vi "Get bronkhorst param from PGserver.vi"(6 "conninfo":T2={"host"="localhost", "port"="5432", "client_encoding"="WIN1251", "dbname"="data", "user"="postgres", "password"=""}, 8 "error in (no error)":errorcluster, 9 "RegParamColumns":string[](array[string])=["instrument_range_max", "auto_value", "alr_value", "output_k", "output_set_time", "group", "process_units", "process_gas", "fcode", "fcode_full", "shortname"], 10 "AIParamTable":string="bronkhorst", 11 "AIParameters":string[](array[string])) -> (0 "error out":errorcluster, 2 "Names table":string[][](array[string]), 3 "Parameters table":dbl[][](array[numeric]))   [LabVIEW 2019, in "control.lvlib"]
uses:
  control.lvlib
  Database/ctl/Coninfo.ctl
  Database/PostgreSQL2LabVIEW/libpqlv/src/PQfinish.vi
  Database/PostgreSQL2LabVIEW/libpqlv/src/PQconnectdb.vi
  Database/PostgreSQL2LabVIEW/libpqlv/src/PQerrorMessage.vi
  Database/PostgreSQL2LabVIEW/libpqlv/src/PQstatus.vi
  <vilib>/dlg_ctls.llb/Space Constant.vi
  Database/Progress.vi
  Database/PostgreSQL.lvlib
  Database/PostgreSQL2LabVIEW/libpqUtility64/libpqutility64.lvlib
  Database/PostgreSQL2LabVIEW/libpqUtility/libpqutility.lvlib
panel:
  out "PQStatus":T1(ring)
  # "group"
  # "process_gas"
  # "fcode"
  # "fcode_full"
  # "shortname"
  # "instrument_range_max"
  # "auto_value"
  # "alr_value"
  # "output_k"
  # "output_set_time"
  # "process_units"
  # "Names"
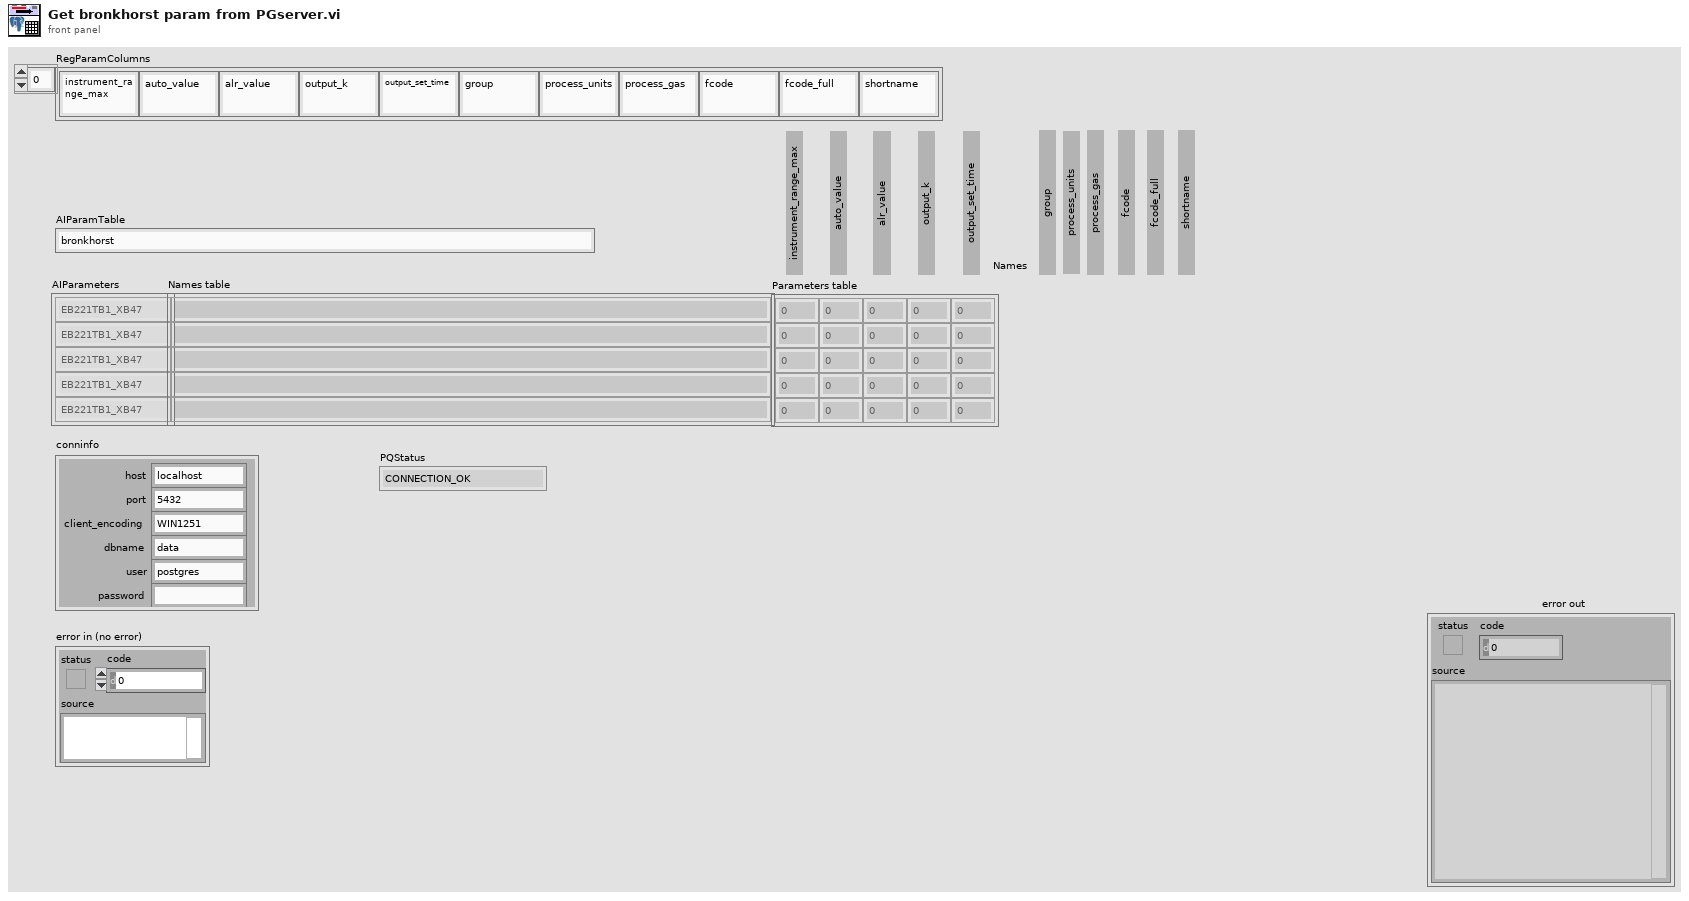
[diagram p1: front panel]
types:
  T1 = enum32{"CONNECTION_OK", "CONNECTION_BAD", "CONNECTION_STARTED", "CONNECTION_MADE", "CONNECTION_AWAITING_RESPONSE", "CONNECTION_AUTH_OK", "CONNECTION_SETENV", "CONNECTION_SSL_STARTUP", "CONNECTION_NEEDED"}
  T2 = typedef "PostgreSQL.lvlib/Coninfo.ctl" = cluster{"host":string, "port":string, "client_encoding":string, "dbname":string, "user":string, "password":string}
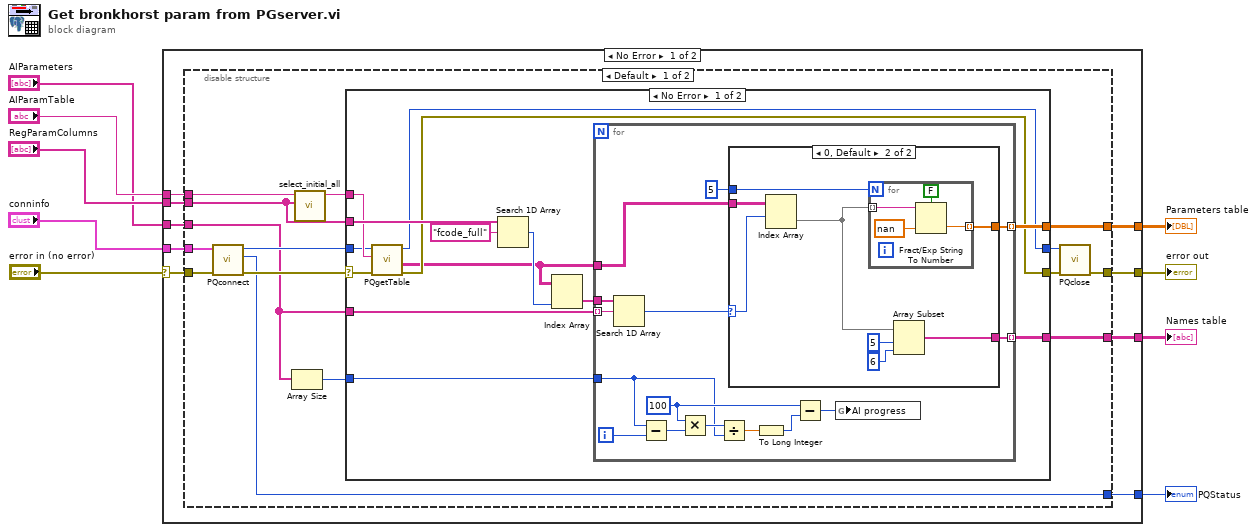
[diagram p0: block diagram]
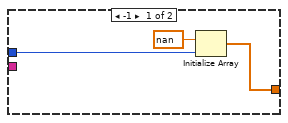
[diagram p2: hidden frame]
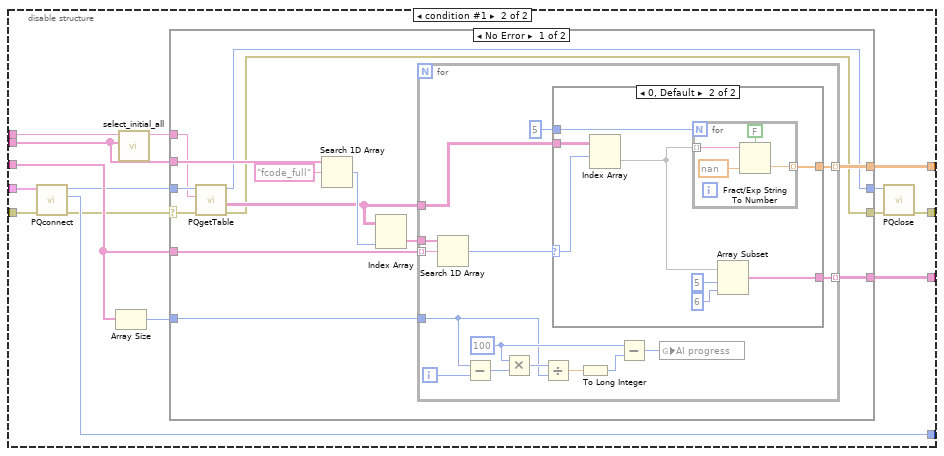
[diagram p4: hidden frame]
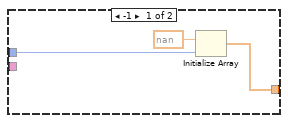
[diagram p5: hidden frame]
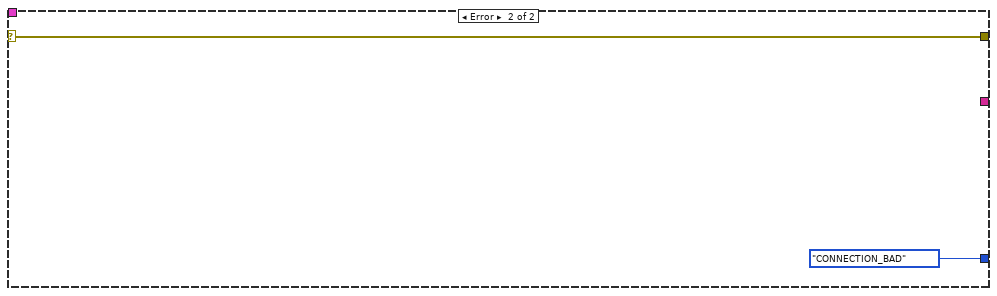
[diagram p7: hidden frame]
diagram:
  n1 = case shown="No Error" "error in (no error)" {
    selector: "error in (no error)" -> [w17 w142]
    tunnel: [w12 w142] -> w9
    tunnel: [w13 _] -> w8
    tunnel: [w11 _] -> w7
    tunnel: "RegParamColumns" -> [w15 _]
    tunnel: "conninfo" -> [w18 _]
    tunnel: "AIParamTable" -> [w16 _]
    tunnel: "AIParameters" -> [w14 _]
    tunnel: [w10 T1."CONNECTION_BAD" ("PQStatus")] -> w1
    frame No Error {
      n2 = disable-structure shown="Default" {
        disable-tunnel: [w22 w80] -> w12
        disable-tunnel: [w27 w88] -> w13
        disable-tunnel: [w26 w89] -> w11
        disable-tunnel: w15 -> [w19 w91]
        disable-tunnel: w18 -> [w30 w87]
        disable-tunnel: w16 -> [w21 w92]
        disable-tunnel: w14 -> [w28 w90]
        disable-tunnel: w17 -> [w29 w86]
        disable-tunnel: [w25 w84] -> w10
        frame condition #0 (active) {
          n3 = call "PQconnect.vi"("error in (no error)"=w29, "conninfo"=w30) -> ("error out"=w33:errorcluster, "PQStatus"=w25:T1, "conn"=w32:u32)  [unwired: 7 in]
          n4 = Array Size(array=w28) -> (size(s)=w31:i32)
          n5 = call "select_initial_all.vi"("Column table"=w19, "table"=w21) -> ("parameters"=w20:string)  [unwired: 8 in, 1 out]
          n6 = case shown="No Error" w33 {
            selector: w33 -> [w40 w79]
            tunnel: w28 -> [w34 _]
            tunnel: [w47 _] -> w27
            tunnel: [w46 _] -> w26
            tunnel: w31 -> [w45 _]
            tunnel: w32 -> [w38 w78]
            tunnel: w20 -> [w39 _]
            tunnel: [w37 w79] -> w23
            tunnel: [w36 w78] -> w24
            tunnel: w19 -> [w41 _]
            frame No Error {
              n7 = call "PQgetTable.vi"("error in"=w40, "query"=w39, "conn"=w38) -> ("error out"=w37:errorcluster, "Data"=w35:string[][], "conn_out"=w36:u32)  [unwired: 4 in, 2 out]
              n8 = Search 1D Array(1D array=w41, element="fcode_full" ("table")) -> (index of element=w43:i32)  [unwired: 1 in]
              n9 = Index Array(array=w35, index (col)=w43) -> (element=w42:string[])  [unwired: 1 in]
              n10 = for {
                tunnel: [w62] -> w46 mode=indexing
                tunnel: [w61] -> w47 mode=indexing
                tunnel: w45 -> [w53]
                tunnel: w42 -> [w51]
                tunnel: w35 -> [w50]
                tunnel: w34 -> [w49] mode=indexing
                i -> [w54]
                w58 = 100 ("y")
                n11 = Search 1D Array(1D array=w51, element=w49) -> (index of element=w48:i32)  [unwired: 1 in]
                n12 = Subtract(x=w53, y=w54) -> (x-y=w57:i32)
                n13 = Multiply(x=w58, y=w57) -> (x*y=w60:i32)
                n14 = Divide(x=w60, y=w53) -> (x/y=w56:dbl)
                n15 = case shown="0, Default" w48 {
                  selector: w48 -> [_ w68]
                  tunnel: [w64 w67] -> w61
                  tunnel: 5 ("y") -> [w63 w71]
                  tunnel: w50 -> [_ w70]
                  tunnel: [_ w72] -> w62
                  frame -1 {
                    n16 = Initialize Array(nan, w63) -> (w64:dbl[])
                  }
                  frame 0, Default {
                    n17 = Index Array(array=w70, index (row)=w68) -> (element=w69:string[])  [unwired: 1 in]
                    n18 = for {
                      N: w71 -> [_]
                      tunnel: w69 -> [w76] mode=indexing
                      tunnel: [w75] -> w67 mode=indexing
                      n19 = Fract/Exp String To Number(use system decimal point (T)=FALSE, string=w76, default (0 dbl)=nan) -> (number=w75:dbl)  [unwired: 1 in, 1 out]
                    }
                    n20 = Array Subset(array=w69, index=5 ("length"), length=6) -> (w72:string[])
                  }
                }
                n21 = To Long Integer(number=w56) -> (32bit integer=w55:i32)
                n22 = Subtract(x=w58, y=w55) -> (x-y=w59:i32)
                n23 = global write "Progress.vi" "AI progress"(w59) -> ()
              }
            }
            frame Error {
            }
          }
          n24 = call "PQclose.vi"("error in (no error)"=w23, "conn"=w24) -> ("error out"=w22:errorcluster)  [unwired: 9 in]
        }
        frame condition #1 {
          n25 = call "PQconnect.vi"("error in (no error)"=w86, "conninfo"=w87) -> ("error out"=w83:errorcluster, "PQStatus"=w84:T1, "conn"=w85:u64)  [unwired: 7 in]
          n26 = Array Size(array=w90) -> (size(s)=w94:i32)
          n27 = call "select_initial_all.vi"("Column table"=w91, "table"=w92) -> ("parameters"=w93:string)  [unwired: 8 in, 1 out]
          n28 = case shown="No Error" w83 {
            selector: w83 -> [w99 w140]
            tunnel: w90 -> [w101 _]
            tunnel: [w108 _] -> w88
            tunnel: [w107 _] -> w89
            tunnel: w94 -> [w106 _]
            tunnel: w85 -> [w100 w139]
            tunnel: w93 -> [w98 _]
            tunnel: [w95 w140] -> w82
            tunnel: [w97 w139] -> w81
            tunnel: w91 -> [w102 _]
            frame No Error {
              n29 = call "PQgetTable.vi"("error in"=w99, "query"=w98, "conn"=w100) -> ("error out"=w95:errorcluster, "Data"=w96:string[][], "conn_out"=w97:u64)  [unwired: 4 in, 2 out]
              n30 = Search 1D Array(1D array=w102, element="fcode_full" ("table")) -> (index of element=w104:i32)  [unwired: 1 in]
              n31 = Index Array(array=w96, index (col)=w104) -> (element=w103:string[])  [unwired: 1 in]
              n32 = for {
                tunnel: [w123] -> w107 mode=indexing
                tunnel: [w122] -> w108 mode=indexing
                tunnel: w106 -> [w114]
                tunnel: w103 -> [w112]
                tunnel: w96 -> [w111]
                tunnel: w101 -> [w110] mode=indexing
                i -> [w115]
                w119 = 100 ("y")
                n33 = Search 1D Array(1D array=w112, element=w110) -> (index of element=w109:i32)  [unwired: 1 in]
                n34 = Subtract(x=w114, y=w115) -> (x-y=w118:i32)
                n35 = Multiply(x=w119, y=w118) -> (x*y=w121:i32)
                n36 = Divide(x=w121, y=w114) -> (x/y=w117:dbl)
                n37 = case shown="0, Default" w109 {
                  selector: w109 -> [_ w129]
                  tunnel: [w125 w128] -> w122
                  tunnel: 5 ("y") -> [w124 w132]
                  tunnel: w111 -> [_ w131]
                  tunnel: [_ w133] -> w123
                  frame -1 {
                    n38 = Initialize Array(nan, w124) -> (w125:dbl[])
                  }
                  frame 0, Default {
                    n39 = Index Array(array=w131, index (row)=w129) -> (element=w130:string[])  [unwired: 1 in]
                    n40 = for {
                      N: w132 -> [_]
                      tunnel: w130 -> [w137] mode=indexing
                      tunnel: [w136] -> w128 mode=indexing
                      n41 = Fract/Exp String To Number(use system decimal point (T)=FALSE, string=w137, default (0 dbl)=nan) -> (number=w136:dbl)  [unwired: 1 in, 1 out]
                    }
                    n42 = Array Subset(array=w130, index=5 ("length"), length=6) -> (w133:string[])
                  }
                }
                n43 = To Long Integer(number=w117) -> (32bit integer=w116:i32)
                n44 = Subtract(x=w119, y=w116) -> (x-y=w120:i32)
                n45 = global write "Progress.vi" "AI progress"(w120) -> ()
              }
            }
            frame Error {
            }
          }
          n46 = call "PQclose.vi"("error in (no error)"=w82, "conn"=w81) -> ("error out"=w80:errorcluster)  [unwired: 9 in]
        }
      }
    }
    frame Error {
    }
  }
  "error out" <- w9
  "Parameters table" <- w8
  "Names table" <- w7
  "PQStatus" <- w1
